vi "CPU_MEM_write_mem.vi"(10 "value":u8 format="%02x", 11 "address":u16 format="%.0x") -> ()   [LabVIEW 2018]
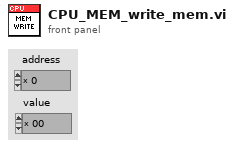
[diagram p1: front panel]
types:
  T1 = enum16{"init", "read DDR", "read PDR", "write DDR", "write PDR"}
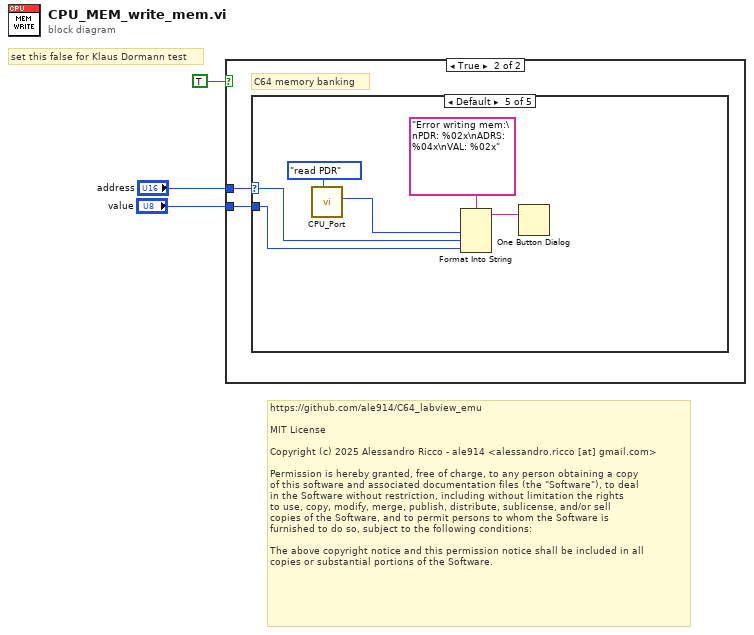
[diagram p0: block diagram]
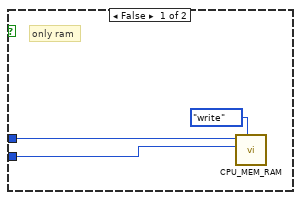
[diagram p2: hidden frame]
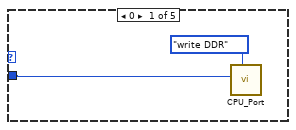
[diagram p3: hidden frame]
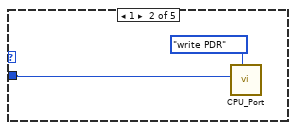
[diagram p4: hidden frame]
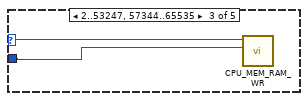
[diagram p5: hidden frame]
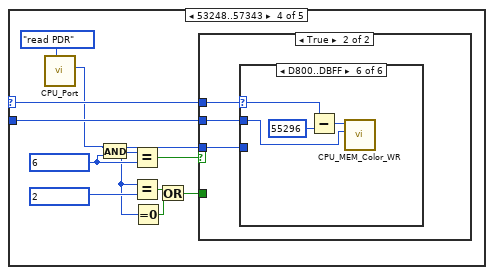
[diagram p6: hidden frame]
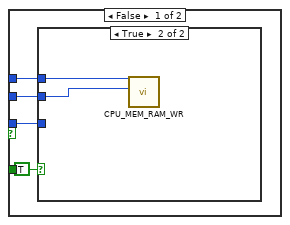
[diagram p7: hidden frame]
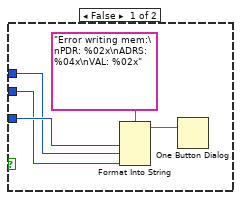
[diagram p8: hidden frame]
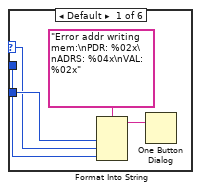
[diagram p9: hidden frame]
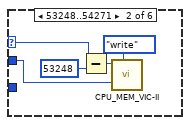
[diagram p10: hidden frame]
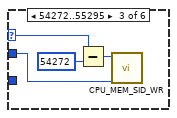
[diagram p11: hidden frame]
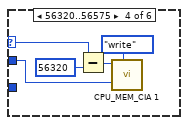
[diagram p12: hidden frame]
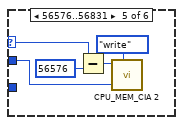
[diagram p13: hidden frame]
diagram:
  # "set this false for Klaus Dormann test"
  # "https://github.com/ale914/C64_labview_emu\n\nMIT License\n\nCopyright (c) 2025 Alessandro Ricco - ale914 <alessandro.ricco [at] gmail.com>\n\nPermission is hereby granted, free of charge, to any person obtaining a copy\nof this software and associated documentation files (the \"Software\"), to deal\nin the Software without restriction, including without limitation the rights\nto use, copy, modify, merge, publish, distribute, sublicense, and/or sell\ncopies of the Software, and to permit persons to whom the Software is\nfurnished to do so, subject to the following conditions:\n\nThe above copyright notice and this permission notice shall be included in all\ncopies or substantial portions of the Software."
  n1 = case shown="True" TRUE {
    tunnel: "address" -> [w5 w8]
    tunnel: "value" -> [w4 w7]
    frame False {
      # "only ram"
      n2 = call "CPU_MEM_RAM.vi"("oper"=enum16{"init", "read", "write"}."write", "value in"=w4, "address"=w5) -> ()  [unwired: 7 in, 2 out]
    }
    frame True {
      # "C64 memory banking"
      n3 = case shown="Default" w8 {
        selector: w8 -> [_ _ w14 w25 w71]
        tunnel: w7 -> [w9 w11 w13 w24 w70]
        frame 0 {
          n4 = call "CPU_Port.vi"("oper"=T1."write DDR", "value in"=w9) -> ()  [unwired: 9 in, 1 out]
        }
        frame 1 {
          n5 = call "CPU_Port.vi"("oper"=T1."write PDR", "value in"=w11) -> ()  [unwired: 9 in, 1 out]
        }
        frame 2..53247, 57344..65535 {
          n6 = call "CPU_MEM_RAM_WR.vi"("value in"=w13, "address"=w14) -> ()  [unwired: 10 in]
        }
        frame 53248..57343 {
          w23 = u8 6 ("y")
          n7 = call "CPU_Port.vi"("oper"=T1."read PDR") -> ("value out"=w21:u8)  [unwired: 10 in]
          n8 = And(x=w21, y=w23) -> (x .and. y?=w17:u8)
          n9 = Equal?(x=w17, y=w23) -> (x = y?=w20:bool)
          n10 = Equal?(x=w17, y=u8 2) -> (x = y?=w18:bool)
          n11 = Equal To 0?(x=w17) -> (x = 0?=w16:bool)
          n12 = Or(x=w18, y=w16) -> (x .or. y?=w15:bool)
          n13 = case shown="True" w20 {
            tunnel: w25 -> [w28 w39]
            tunnel: w24 -> [w27 w38]
            tunnel: w21 -> [w29 w37]
            tunnel: w15 -> [_ _]
            frame False {
              n14 = case shown="True" TRUE {
                tunnel: w29 -> [w32 _]
                tunnel: w28 -> [w31 w36]
                tunnel: w27 -> [w30 w35]
                frame False {
                  n15 = Format Into String(format string="Error writing mem:\nPDR: %02x\nADRS: %04x\nVAL: %02x", w32, w31, w30) -> (resulting string=w33:string)  [unwired: 2 in, 1 out]
                  n16 = One Button Dialog(message=w33) -> ()  [unwired: 1 in, 1 out]
                }
                frame True {
                  n17 = call "CPU_MEM_RAM_WR.vi"("value in"=w35, "address"=w36) -> ()  [unwired: 10 in]
                }
              }
            }
            frame True {
              n18 = case shown="D800..DBFF" w39 {
                selector: w39 -> [w41 w49 w52 w58 w63 w66]
                tunnel: w38 -> [w40 w48 w50 w57 w62 w65]
                tunnel: w37 -> [w42 _ _ _ _ _]
                frame Default {
                  n19 = Format Into String(format string="Error addr writing mem:\nPDR: %02x\nADRS: %04x\nVAL: %02x", w42, w41, w40) -> (resulting string=w43:string)  [unwired: 2 in, 1 out]
                  n20 = One Button Dialog(message=w43) -> ()  [unwired: 1 in, 1 out]
                }
                frame 53248..54271 {
                  n21 = Subtract(x=w49, y=u16 53248 ("address")) -> (x-y=w45:u16)
                  n22 = call "CPU_MEM_VIC-II.vi"("oper"=enum16{"init", "read", "write"}."write", "value in"=w48, "address"=w45) -> ()  [unwired: 7 in, 2 out]
                }
                frame 54272..55295 {
                  n23 = Subtract(x=w52, y=u16 54272 ("address")) -> (x-y=w51:u16)
                  n24 = call "CPU_MEM_SID_WR.vi"("value in"=w50, "address"=w51) -> ()  [unwired: 10 in]
                }
                frame 56320..56575 {
                  n25 = Subtract(x=w58, y=u16 56320 ("address")) -> (x-y=w54:u16)
                  n26 = call "CPU_MEM_CIA 1.vi"("oper"=enum16{"init", "read", "write"}."write", "value in"=w57, "address"=w54) -> ()  [unwired: 7 in, 2 out]
                }
                frame 56576..56831 {
                  n27 = Subtract(x=w63, y=u16 56576 ("address")) -> (x-y=w59:u16)
                  n28 = call "CPU_MEM_CIA 2.vi"("oper"=enum16{"init", "read", "write"}."write", "value in"=w62, "address"=w59) -> ()  [unwired: 8 in, 1 out]
                }
                frame 55296..56319 {
                  n29 = Subtract(x=w66, y=u16 55296 ("address")) -> (x-y=w64:u16)
                  n30 = call "CPU_MEM_Color_WR.vi"("value in"=w65, "address"=w64) -> ()  [unwired: 10 in]
                }
              }
            }
          }
        }
        frame Default {
          n31 = call "CPU_Port.vi"("oper"=T1."read PDR") -> ("value out"=w68:u8)  [unwired: 10 in]
          n32 = Format Into String(format string="Error writing mem:\nPDR: %02x\nADRS: %04x\nVAL: %02x", w68, w71, w70) -> (resulting string=w72:string)  [unwired: 2 in, 1 out]
          n33 = One Button Dialog(message=w72) -> ()  [unwired: 1 in, 1 out]
        }
      }
    }
  }
